vi "Append Text.vi"(8 "error in (no error)":errorcluster, 9 "Style":refnum<class "Style.lvclass">, 10 "Text":string, 11 "xwpfWriter in":refnum<class "xwpfWriter.lvclass">) -> (0 "error out":errorcluster, 3 "xwpfWriter out":refnum<class "xwpfWriter.lvclass">)   [LabVIEW 2017, in "xwpfWriter.lvclass"]
doc: "Appends <b>Text</b> formating as defined by <b>Style</b> after the last paragraph within the document."
uses:
  xwpfWriter.lvclass
  Styles/Style/Style.lvclass
  xwpfWriter.lvclass/xwpfWriter.ctl
  C:/Users/Neo/Desktop/Dev_Tools_BR/LabVIEW_NPOI/src/lib/NPOI 2.1.1/NPOI.OOXML.dll
  lib/NPOI 2.1.1/NPOI.OOXML.dll
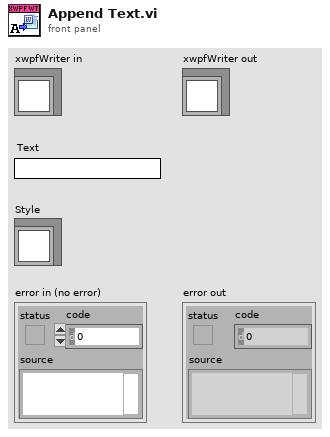
[diagram p1: front panel]
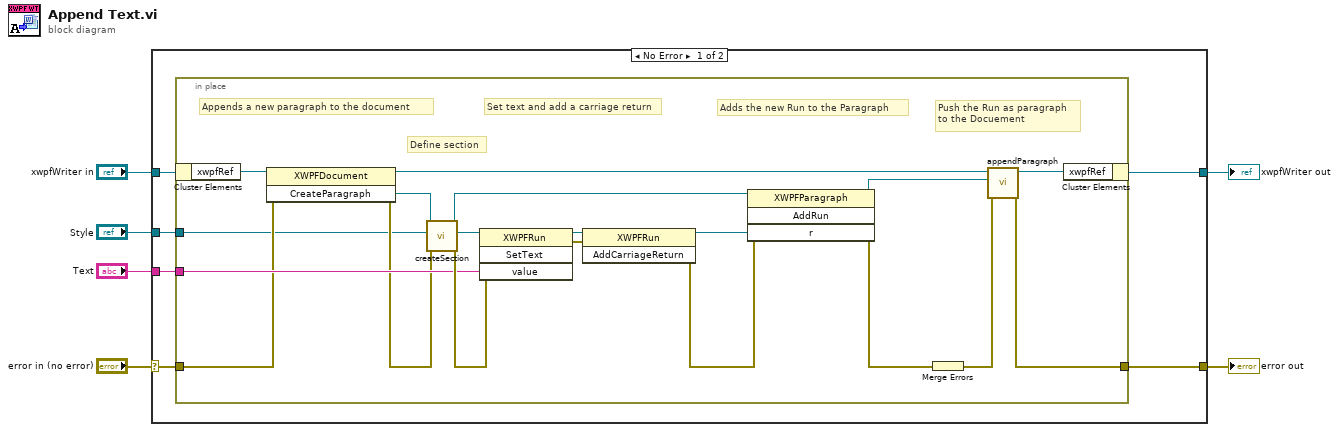
[diagram p0: block diagram]
diagram:
  n1 = case shown="No Error" "error in (no error)" {
    selector: "error in (no error)" -> [w10 w33]
    tunnel: [w7 w33] -> w5
    tunnel: [w12 w32] -> w3
    tunnel: "xwpfWriter in" -> [w11 w32]
    tunnel: "Style" -> [w9 _]
    tunnel: "Text" -> [w8 _]
    frame No Error {
      n2 = in-place {
        in-place-border: w10 -> [w20]
        in-place-border: w9 -> [w15]
        in-place-border: w8 -> [w23]
        in-place-border: [w17] -> w7
        # "Push the Run as paragraph\nto the Docuement"
        # "Adds the new Run to the Paragraph"
        # "Define section"
        # "Set text and add a carriage return"
        # "Appends a new paragraph to the document"
        n3 = in-place-cluster #1(w11) -> ("xwpfRef"=w31:refnum<k24>)
        n4 = invoke class="XWPFDocument" method="CreateParagraph"(reference=w31, error in=w20) -> (reference out=w29:refnum<k24>, error out=w19:errorcluster, "CreateParagraph"=w30:refnum<k24>)  [unwired: 1 in]
        n5 = call "createSection.vi"("error in (no error)"=w19, "Style"=w15, "Paragraph in"=w30) -> ("error out"=w24:errorcluster, "Section out"=w25:refnum<k24>, "Paragraph out"=w16:refnum<k24>)  [unwired: 6 in]
        n6 = invoke class="XWPFRun" method="SetText"(reference=w25, error in=w24, "value"=w23) -> (reference out=w26:refnum<k24>, error out=w27:errorcluster)  [unwired: 1 in, 2 out]
        n7 = invoke class="XWPFRun" method="AddCarriageReturn"(reference=w26, error in=w27) -> (reference out=w13:refnum<k24>, error out=w21:errorcluster)  [unwired: 1 in, 1 out]
        n8 = invoke class="XWPFParagraph" method="AddRun"(reference=w16, error in=w21, "r"=w13) -> (reference out=w14:refnum<k24>, error out=w22:errorcluster)  [unwired: 1 in, 2 out]
        n9 = Merge Errors(w22) -> (w18:errorcluster)
        n10 = call "appendParagraph.vi"("error in (no error)"=w18, "paragraph"=w14, "XWPFDocuement in"=w29) -> ("error out"=w17:errorcluster, "XWPFDocuement out"=w28:refnum<k24>)  [unwired: 7 in]
        n11 = in-place-cluster #1("xwpfRef"=w28) -> (w12:refnum<class "xwpfWriter.lvclass">)
      }
    }
    frame Error {
    }
  }
  "error out" <- w5
  "xwpfWriter out" <- w3
